vi "GetText.vi"(8 "error in (no error)":errorcluster, 10 "MenuItem":refnum<class "MGI_MenuItem.lvclass">, 11 "NotifyIcon in":refnum<class "MGI_TrayIcon.lvclass">) -> (0 "error out":errorcluster, 2 "Text":string, 3 "NotifyIcon out":refnum<class "MGI_TrayIcon.lvclass">)   [LabVIEW 2016, in "MGI_TrayIcon.lvclass"]
doc: "Gets the Text from the menu. \n\nThis is different that using the property node on the MenuItem because this will access the actual menu and query the field.\n\nAuthored by Derek E. Trepanier\nsupport@mooregoodideas.com\nwww.mooregoodideas.com\n\nCopyright (c) 2012, Moore Good Ideas, Inc.\n\nAll rights reserved.\n\nRedistribution and use in source and binary forms, with or without modification, are permitted provided that the following conditions are met:\n\n * Redistributions of source code must retain the above copyright notice, this list of conditions and the following disclaimer.\n * Redistributions in binary form must reproduce the above copyright notice, this list of conditions and the following disclaimer in the documentation and/or other materials provided with the distribution.\n * Neither the name of Moore Good Ideas, Inc. nor the names of its contributors may be used to endorse or promote products derived from this software without specific prior written permission.\n\nTHIS SOFTWARE IS PROVIDED BY THE COPYRIGHT HOLDERS AND CONTRIBUTORS \"AS IS\" AND ANY EXPRESS OR IMPLIED WARRANTIES, INCLUDING, BUT NOT LIMITED TO, THE IMPLIED WARRANTIES OF MERCHANTABILITY AND FITNESS FOR A PARTICULAR PURPOSE ARE DISCLAIMED. IN NO EVENT SHALL THE COPYRIGHT OWNER OR CONTRIBUTORS BE LIABLE FOR ANY DIRECT, INDIRECT, INCIDENTAL, SPECIAL, EXEMPLARY, OR CONSEQUENTIAL DAMAGES (INCLUDING, BUT NOT LIMITED TO, PROCUREMENT OF SUBSTITUTE GOODS OR SERVICES; LOSS OF USE, DATA, OR PROFITS; OR BUSINESS INTERRUPTION) HOWEVER CAUSED AND ON ANY THEORY OF LIABILITY, WHETHER IN CONTRACT, STRICT LIABILITY, OR TORT (INCLUDING NEGLIGENCE OR OTHERWISE) ARISING IN ANY WAY OUT OF THE USE OF THIS SOFTWARE, EVEN IF ADVISED OF THE POSSIBILITY OF SUCH DAMAGE."
uses:
  <userlib>/_MGI/Menu Building/MenuTypes/TrayIcon/MGI_TrayIcon.lvclass
  <userlib>/_MGI/Menu Building/MenuItem/MGI_MenuItem.lvclass
  System.Windows.Forms
  <userlib>/_MGI/Menu Building/MenuItem/Read Full Tag.vi
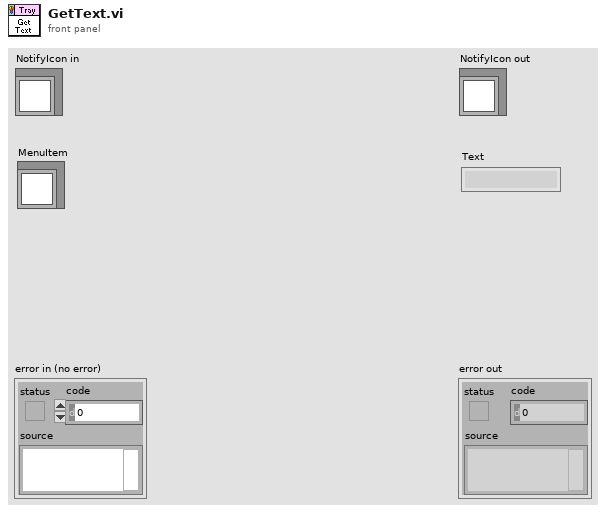
[diagram p1: front panel]
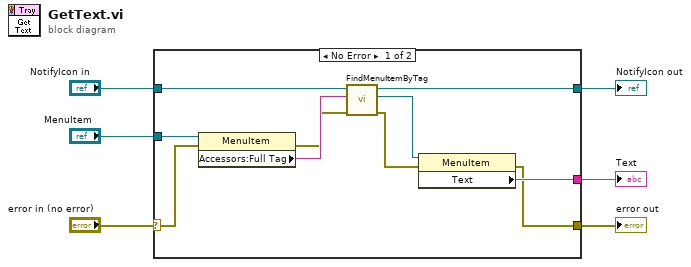
[diagram p0: block diagram]
diagram:
  n1 = case shown="No Error" "error in (no error)" {
    selector: "error in (no error)" -> [w11 w18]
    tunnel: [w7 w18] -> w2
    tunnel: [w9 w17] -> w3
    tunnel: "NotifyIcon in" -> [w16 w17]
    tunnel: "MenuItem" -> [w15 _]
    tunnel: [w10 _] -> w1
    frame No Error {
      n2 = property class="MenuItem"(reference=w15, error in=w11) -> (error out=w12:errorcluster, "Accessors:Full Tag"=w14:string)  [unwired: 1 out]
      n3 = call <userlib>:"FindMenuItemByTag.vi"("error in (no error)"=w12, "Full Tag"=w14, "NotifyIcon in"=w16) -> ("error out"=w8:errorcluster, "Menu Item"=w13:refnum<k24>, "NotifyIcon out"=w9:refnum<class "MGI_TrayIcon.lvclass">)  [unwired: 6 in]
      n4 = property class="MenuItem"(reference=w13, error in=w8) -> (error out=w7:errorcluster, "Text"=w10:string)  [unwired: 1 out]
    }
    frame Error {
    }
  }
  "error out" <- w2
  "NotifyIcon out" <- w3
  "Text" <- w1
